vi "test_LogLevelSettings_DebugEventInfoSink_EventNotLogged.vi"(8 "error in (no error)":errorcluster, 11 "TestCase in":refnum<class "TestDataSink.lvclass">) -> (0 "error out":errorcluster, 3 "TestCase out":refnum<class "TestDataSink.lvclass">)   [LabVIEW 2017, in "TestDataSink.lvclass"]
uses:
  TestDataSink.lvclass
  Source/Composed Log/Types/Log Level.ctl
  Source/LVQueue Sink/LVQueue Sink.lvclass/LVQueue Sink.ctl
  Source/Composed Log/LoggerReference/LoggerReference.lvclass/LoggerReference.ctl
  80d186c3-302b-4919-999c-927c3d77a8df.vi
  80d186c3-302b-4919-999c-927c3d77a8df.vi/1bdb29c5-eb28-44dc-aaca-f6f98509e224.vi
  Source/Composed Log/LoggerReference/Return Aggregate Queues.vi
  Source/Composed Log/LoggerReference/Add Aggregate Log.vi
  80d186c3-302b-4919-999c-927c3d77a8df.vi/1bdb29c5-eb28-44dc-aaca-f6f98509e224.vi/54cee511-4499-4928-8e3d-b813441b8715.vi
  Source/Composed Log/LoggerReference/Log.vi
  Source/Composed Log/LoggerReference/Send Add Sink.vi
  Source/Composed Log/LoggerReference/Remove Stale Logs.vi
  Source/LVQueue Sink/LVQueue Sink.lvclass
  C:/CS/Internal/LabVIEW/Logger/Source/Composed Log/Log Sink/Log Sink.lvclass
  Source/Composed Log/Application Logger/Launch Worker Loop.vi
  Source/Composed Log/LoggerReference/Initialize Logger Instance.vi
  Source/Composed Log/Singleton Event Log/Logger Queue FGV.vi
  Source/Composed Log/IErrorFormat/IErrorFormat.lvclass
  Source/Composed Log/LoggerReference/LoggerReference.lvclass
  Source/Composed Log/Log Sink/Log Sink.lvclass
  Source/Composed Log/Singleton Event Log/Singleton Event Log.lvlib
  Source/Composed Log/Composed Log.lvlib
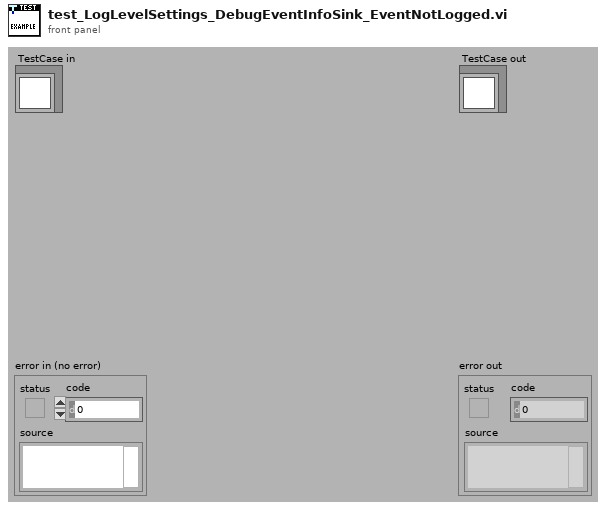
[diagram p1: front panel]
types:
  T1 = typedef "Composed Log.lvlib/Log Level.ctl" = enum16{"Debug", "Info", "Warning", "Error", "Critical"}
  T2 = typedef "Composed Log.lvlib/Log Packet.ctl" = cluster{"Data To Log":string, "Source":string, "Event Level":T1, "Event Time":timestamp}
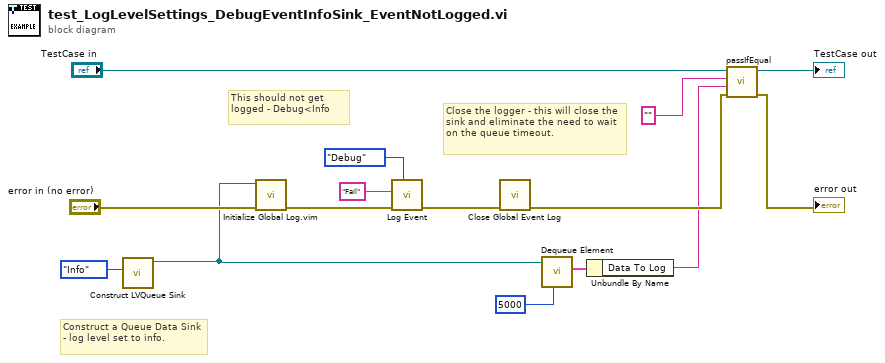
[diagram p0: block diagram]
diagram:
  # "Close the logger - this will close the sink and eliminate the need to wait on the queue timeout."
  # "Construct a Queue Data Sink - log level set to info."
  # "This should not get logged - Debug<Info"
  n1 = call "Construct LVQueue Sink.vi"("LogLevel"=Log_Level."Info") -> ("LVQueue Sink out"=w11:refnum<class "LVQueue Sink.lvclass">)  [unwired: 9 in, 1 out]
  n2 = call "Initialize Global Log.vim"("error in (no error)"="error in (no error)", "Log Sink(s)"=w11) -> ("error out"=w3:errorcluster)  [unwired: 8 in, 1 out]
  n3 = call "Log Event.vi"("Event Level"=Log_Level."Debug", "error in (no error)"=w3, "Data To Log"="Fail") -> ("error out"=w2:errorcluster)  [unwired: 8 in]
  n4 = call "Close Global Event Log.vi"("error in (no error)"=w2) -> ("error out"=w8:errorcluster)  [unwired: 10 in]
  n5 = call "Dequeue Element.vi"("timeout in ms (-1)"=5000, "LVQueue Sink in"=w11) -> ("Log Packet"=w7:T2)  [unwired: 6 in, 3 out]
  n6 = Unbundle By Name(w7) -> ("Data To Log"=w5:string)
  n7 = call-dynamic "passIfEqual.vi"("error in (no error)"=w8, "y"=w5, "x"="" ("Data To Log"), "TestCase in"="TestCase in") -> ("error out"=→"error out":errorcluster, "TestCase out"=→"TestCase out":refnum<class "TestDataSink.lvclass">)  [unwired: 6 in]
